vi "compareArrayDataHold.vi"(9 "B":variant, 10 "A":variant) -> (1 "Value":u16, 2 "BitChange":i32)   [LabVIEW 2014]
panel:
  in  "HoldingChange":u16[](array[numeric])
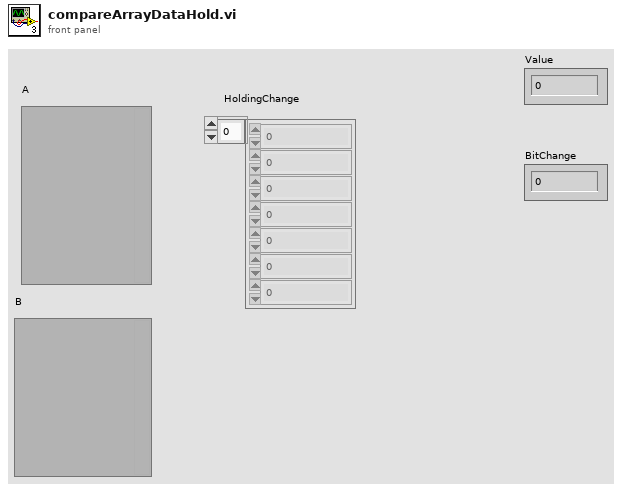
[diagram p1: front panel]
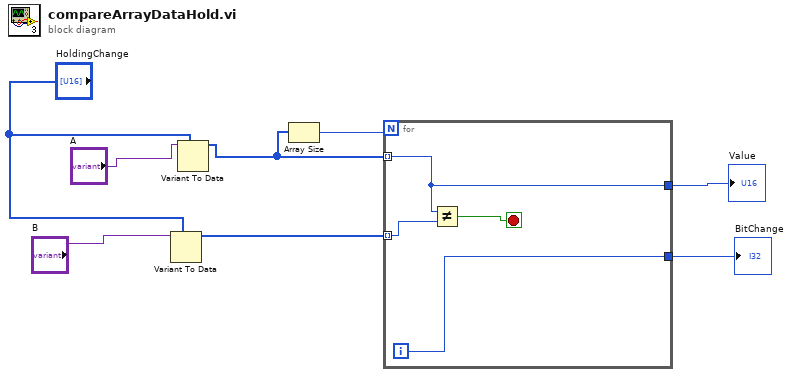
[diagram p0: block diagram]
diagram:
  n1 = Variant To Data(type="HoldingChange", Variant="B") -> (data=w6:u16[])  [unwired: 1 in, 1 out]
  n2 = Variant To Data(type="HoldingChange", Variant="A") -> (data=w5:u16[])  [unwired: 1 in, 1 out]
  n3 = Array Size(array=w5) -> (size(s)=w4:i32)
  n4 = for {
    N: w4 -> [_]
    tunnel: w5 -> [w9] mode=indexing
    tunnel: w6 -> [w12] mode=indexing
    tunnel: [w10] -> w3
    tunnel: [w9] -> w1
    i -> [w10]
    stop <- w11 stop-if-true
    n5 = Not Equal?(x=w9, y=w12) -> (x != y?=w11:bool)
  }
  "BitChange" <- w3
  "Value" <- w1
